vi "reCalibratePlatforms_allButOne.vi"(6 "mazeDirection":string, 8 "error in (no error)":errorcluster, 10 "Current location":dbl) -> (0 "error out":errorcluster)   [LabVIEW 2017]
doc: "The load cells output a voltage even when no weight is present on the platform. This needs to be measured so that it can be subtracted from subsequent measurements of platform load. The VI will output a spreadsheet saved in the current folder."
uses:
  <vilib>/Utility/error.llb/DialogType.ctl
  <vilib>/Utility/file.llb/Write Delimited Spreadsheet (string).vi
  <vilib>/Utility/file.llb/Write Delimited Spreadsheet (DBL).vi
panel:
  out "message":string=" INSTRUCTIONS:\r\rNormal Use:  When using subVIs that incorporate the error in/error out (or error I/O) structure, place this handler where you want to inform the user of an error, typically at the end of the I/O data path, as the last action of the program.  If the error in error? is ERROR, the handler creates a message describing the error and its source.  If the type of dialog = 1 (default), the message is displayed to the user, who can only acknowedge it.  If the type = 2, the user can acknowledge the message or abort execution; aborting a program with active I/O is not recommended.  If the type = 0, no message is displayed; this is used to process the error programmatically, and the error out cluster elements are wired to individual terminals for that reason.  \r\rOther Use:\n\r\nlocal testing.  To test the error code of a subVI or function that does not have the error I/O structure, you can wire its error code and a source string to the local error code and error source inputs.  If error in error? indicates no error and error code is not equal to 0, the local code and source are substituted for the error in values, and error? is set TRUE (ERROR)."
  out "source out":string
  out "code out":i32 format="%0.0f"
  out "error?":bool
  in  "type of dialog (OK msg:1)":T1=1 items=["no dialog", "OK message", "continue or stop message", "OK message + warnings", "continue/stop + warnings"]
  in  "error source (\" \")":string
  in  "error code (no error:0)":i32 format="%0.0f"
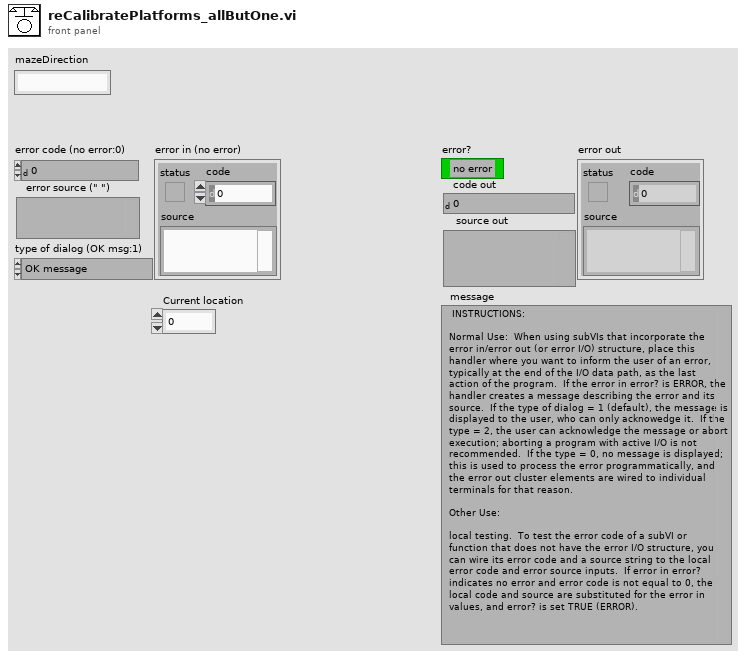
[diagram p1: front panel]
types:
  T1 = typedef "DialogType.ctl" = u16
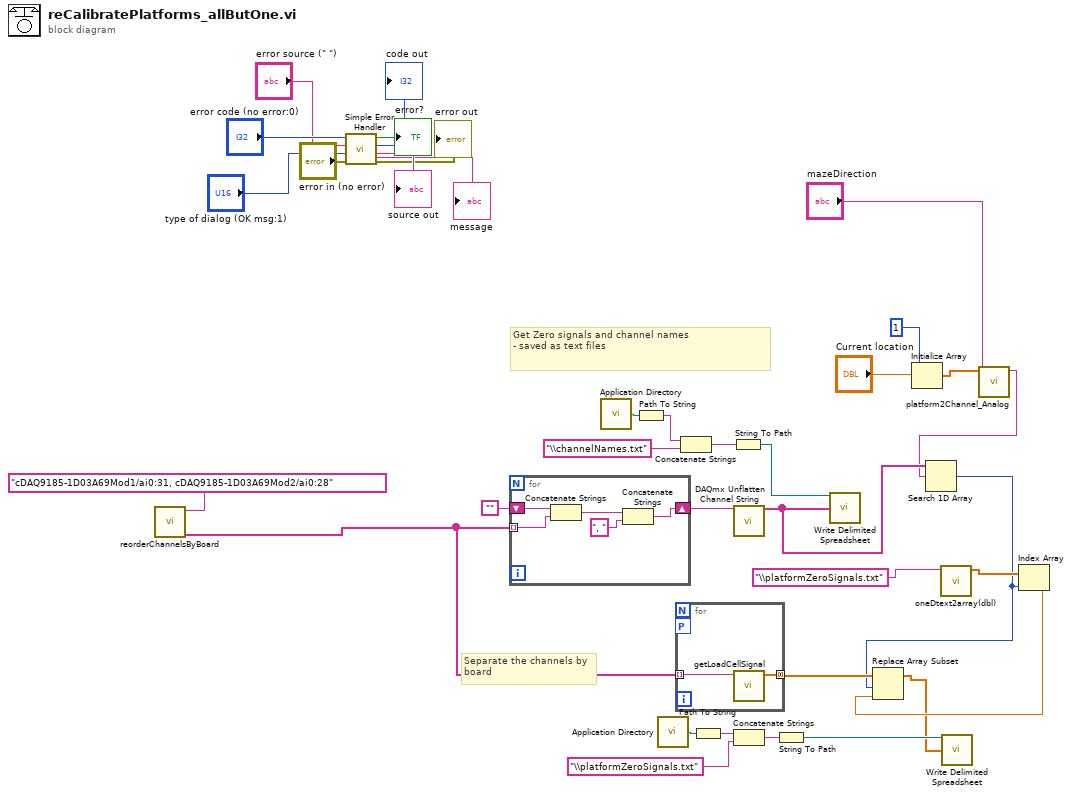
[diagram p0: block diagram]
diagram:
  # "Separate the channels by\nboard"
  # "Get Zero signals and channel names \n- saved as text files"
  n1 = call "reorderChannelsByBoard.vi"("DAQmx \nPhysical Channel"=tag "cDAQ9185-1D03A69Mod1/ai0:31, cDAQ9185-1D03A69Mod2/ai0:28" ("DAQmx \nPhysical Channel")) -> ("Separated inputs\nas strings"=w25:string[])  [unwired: 8 in, 2 out]
  n2 = call <vilib>:"Simple Error Handler.vi"("error code (no error:0)"="error code (no error:0)", "error source (\" \")"="error source (\" \")", "type of dialog (OK msg:1)"="type of dialog (OK msg:1)", "error in (no error)"="error in (no error)") -> ("error?"=→"error?":bool, "code out"=→"code out":i32, "source out"=→"source out":string, "error out"=→"error out":errorcluster, "message"=→"message":string)  [unwired: 1 in]
  n3 = for {
    shift-right: [w39] -> w23
    shift-left: "" -> [w40]
    tunnel: w25 -> [w36] mode=indexing
    n4 = Concatenate Strings(w40, w36) -> (w38:string)
    n5 = Concatenate Strings(w38, ", ") -> (w39:string)
  }
  n6 = call <vilib>:"Application Directory.vi"() -> ("Application Directory"=w21:path)
  n7 = Path To String(path=w21) -> (string=w20:string)
  n8 = call <vilib>:"Application Directory.vi"() -> ("Application Directory"=w16:path)
  n9 = for {
    workers-P: _ -> [_]
    tunnel: [w41] -> w6 mode=concatenating
    tunnel: w25 -> [w42] mode=indexing
    n10 = call "getLoadCellSignal.vi"("DAQmx Physical Channel"=w42) -> ("load cell\nsignal"=w41:dbl[])  [unwired: 10 in]
  }
  n11 = Concatenate Strings(w20, "\\channelNames.txt") -> (w19:string)
  n12 = Path To String(path=w16) -> (string=w15:string)
  n13 = String To Path(string=w19) -> (path=w18:path)
  n14 = call <vilib>:"DAQmx Unflatten Channel String.vi"("names in"=w23) -> ("names out"=w10:string[])  [unwired: 13 in, 1 out]
  n15 = Concatenate Strings(w15, "\\platformZeroSignals.txt") -> (w14:string)
  n16 = String To Path(string=w14) -> (path=w13:path)
  n17 = call-poly <vilib>:"Write Delimited Spreadsheet.vi"("file path (dialog if empty)"=w18, "1D data"=w10) -> ()  [unwired: 12 in, 2 out]
  n18 = Initialize Array("Current location", 1 ("dimension size")) -> (w11:dbl[])
  n19 = call "oneDtext2array(dbl).vi"("String"="\\platformZeroSignals.txt") -> ("array"=w7:dbl[])  [unwired: 10 in]
  n20 = call "platform2Channel_Analog.vi"("mazeDirection"="mazeDirection", "platforms"=w11) -> ("DAQmx Channel"=w9:string)  [unwired: 9 in]
  n21 = Search 1D Array(1D array=w10, element=w9) -> (index of element=w5:i32)  [unwired: 1 in]
  n22 = Index Array(array=w7, index=w5) -> (element=w4:dbl)
  n23 = Replace Array Subset(array=w6, new element=w4, index=w5) -> (w3:dbl[])
  n24 = call-poly <vilib>:"Write Delimited Spreadsheet.vi"("file path (dialog if empty)"=w13, "1D data"=w3) -> ()  [unwired: 12 in, 2 out]
